vi "Rising Edge Detector.vi"(7 "signal":bool) -> (8 "edge detected":bool)   [LabVIEW 2012]
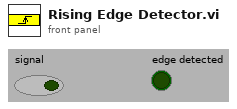
[diagram p1: front panel]
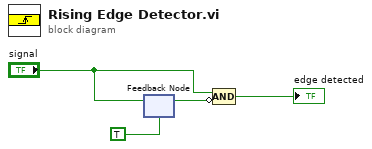
[diagram p0: block diagram]
diagram:
  n1 = feedback-in #1("signal") -> ()
  n2 = feedback #1(TRUE) -> (w3:bool)
  n3 = Compound Arithmetic op=AND("signal", invert w3) -> (→"edge detected":bool)
